vi "Write Items ref.vi"(8 "error in (no error)":errorcluster, 10 "Items ref":refnum<vi>, 11 "Sequence Element in":refnum<class "Sequence Element.lvclass">) -> (0 "error out":errorcluster, 3 "Sequence Element out":refnum<class "Sequence Element.lvclass">)   [LabVIEW 2016, in "Sequence Element.lvclass"]
uses:
  Sequence Element.lvclass
  Sequence Element.lvclass/Sequence Element.ctl
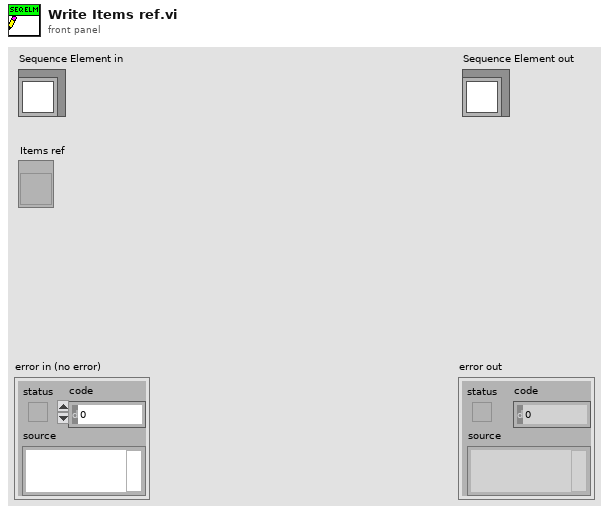
[diagram p1: front panel]
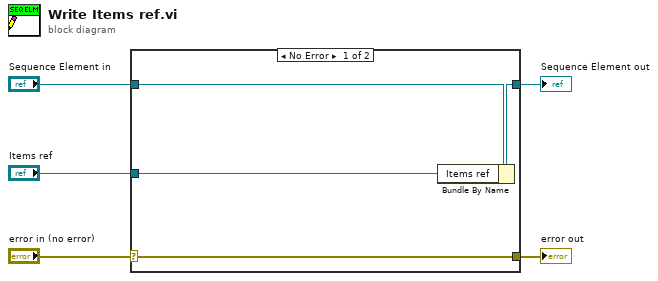
[diagram p0: block diagram]
diagram:
  n1 = case shown="No Error" "error in (no error)" {
    selector: "error in (no error)" -> [w9 w10]
    tunnel: [w9 w10] -> w4
    tunnel: [w7 w11] -> w2
    tunnel: "Sequence Element in" -> [w8 w11]
    tunnel: "Items ref" -> [w6 _]
    frame No Error {
      n2 = Bundle By Name(cluster=w8, "Items ref"=w6) -> (w7:refnum<class "Sequence Element.lvclass">)
    }
    frame Error {
    }
  }
  "error out" <- w4
  "Sequence Element out" <- w2
